vi "staticRFChannelUpdate.vi"(8 "error in (no error)":errorcluster, 10 "staticChannelUpdate":T1, 11 "HWController in":refnum<class "HWController.lvclass">) -> (0 "error out":errorcluster, 3 "HWController out":refnum<class "HWController.lvclass">)   [LabVIEW 2009, in "Hardware.lvlib" / "HWControllers.lvlib" / "HWController.lvclass"]
uses:
  HWController.lvclass
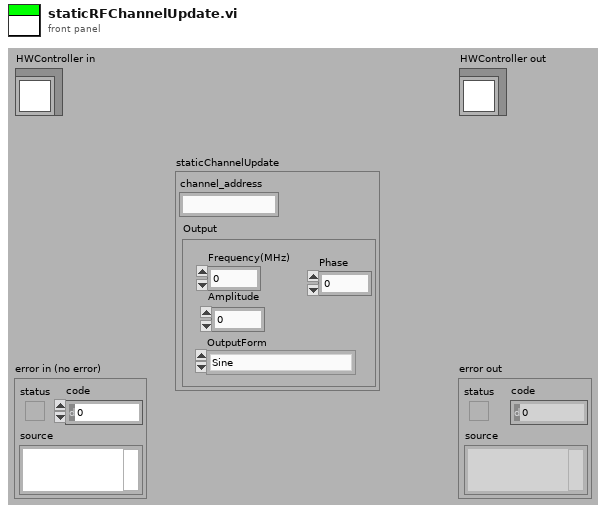
[diagram p1: front panel]
types:
  T1 = cluster{"channel_address":string, "Output":cluster{"Frequency(MHz)":dbl, "Amplitude":dbl, "Phase":dbl, "OutputForm":enum16{"Sine", "Square", "Triangle", "Arbitrary"}}}
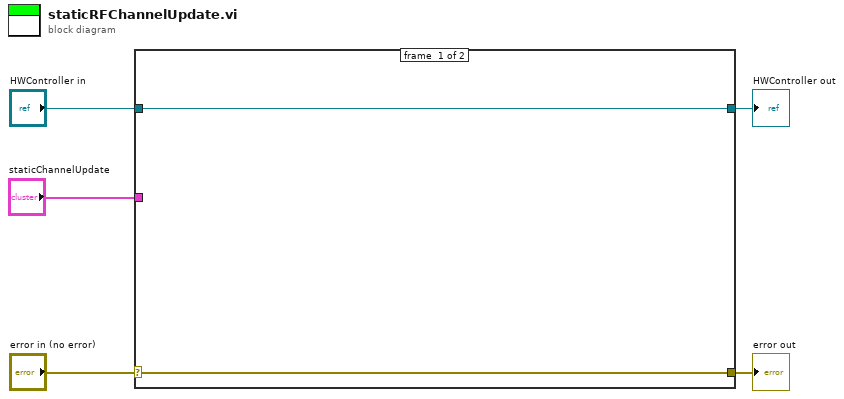
[diagram p0: block diagram]
diagram:
  n1 = case shown="No Error" "error in (no error)" {
    selector: "error in (no error)" -> [w6 w9]
    tunnel: [w6 w9] -> w4
    tunnel: [w7 w8] -> w2
    tunnel: "HWController in" -> [w7 w8]
    tunnel: "staticChannelUpdate" -> [_ _]
    frame #0 {
    }
    frame #1 {
    }
  }
  "error out" <- w4
  "HWController out" <- w2
